vi "Dispose.vi"(8 "error in (no error)":errorcluster, 11 "ConcreteProductA in":refnum<class "ConcreteProductA.lvclass">) -> (0 "error out":errorcluster)   [LabVIEW 2020, in "FactoryMethod.lvlib" / "ConcreteProductA.lvclass"]
uses:
  ConcreteProductA.lvclass
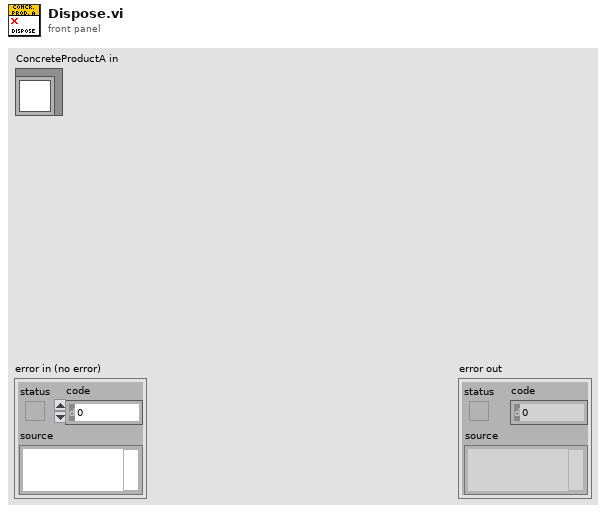
[diagram p1: front panel]
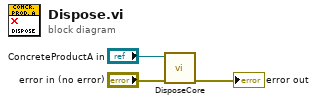
[diagram p0: block diagram]
diagram:
  n1 = call-dynamic "DisposeCore.vi"("error in (no error)"="error in (no error)", "ConcreteProductA in"="ConcreteProductA in") -> ("error out"=→"error out":errorcluster)  [unwired: 8 in, 1 out]
